vi "FTW-Example-ExpressionEvaluation.vi"() -> ()   [LabVIEW 2013]
uses:
  src/core/expression/FTW-Expr-BooleanExpressionResult.ctl
panel:
  out "All expectations satisfied?":bool=TRUE
  out "Tokenized Outputs":T2(array[cluster]) {"Compile Time" format="%.6fsec"; "Execute Time" format="%.6fsec"}
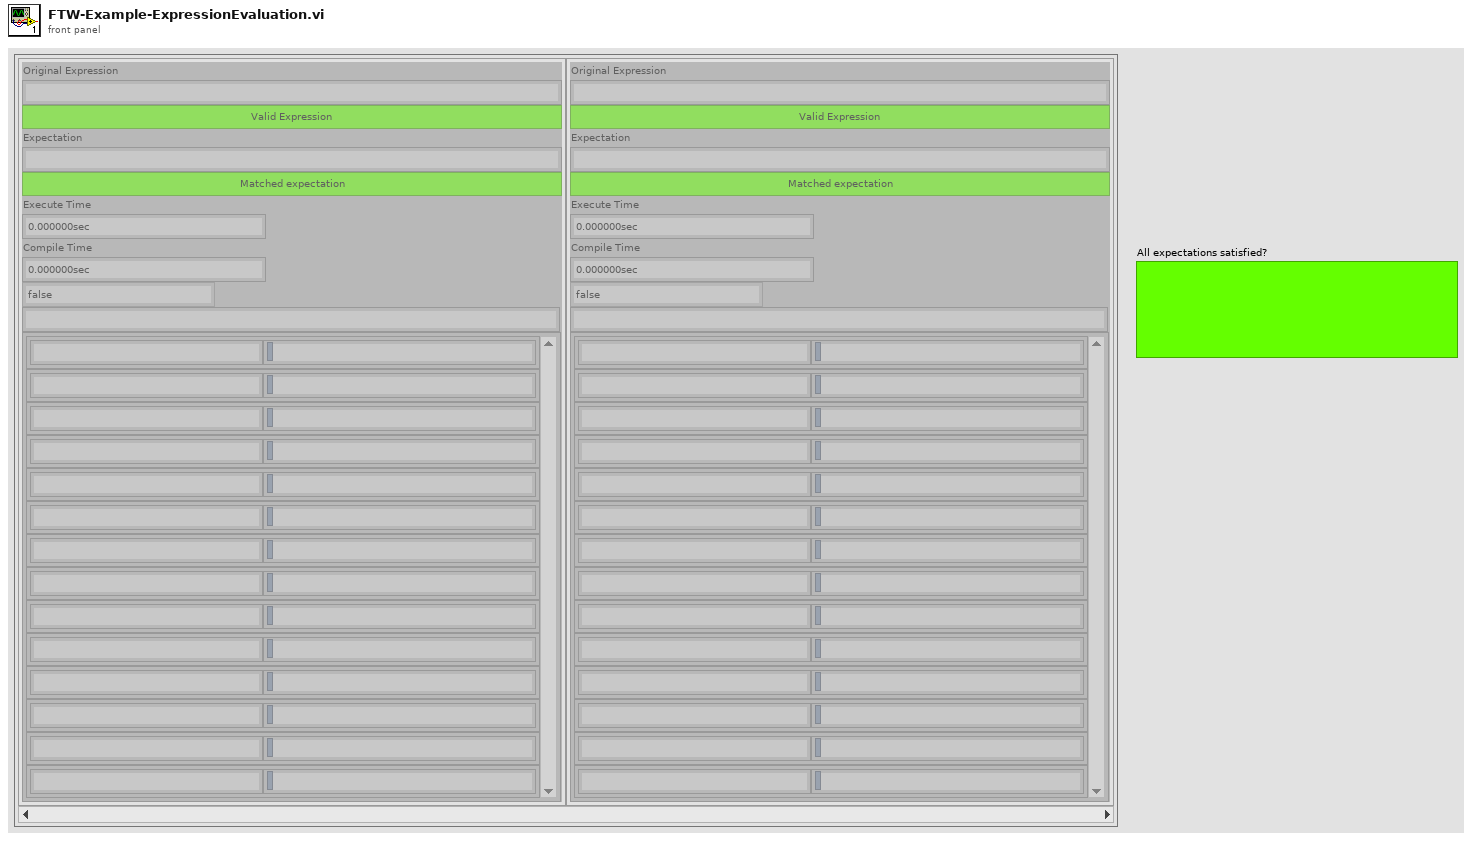
[diagram p1: front panel]
types:
  T1 = typedef "FTW-Expr-BooleanExpressionResult.ctl" = enum16{"false", "true", "inconclusive"}
  T2 = cluster{"Original Expression":string, "Valid?":bool, "Expectation":string, "Expectation satisfied?":bool, "Execute Time":dbl, "Compile Time":dbl, "Result":T1, "Error":string, "Tokens":cluster{string, string}[]}[]
  T3 = cluster{"Expression":string, "Expectation":string}[]
  T4 = cluster{"Expression":string, "Status OK?":bool, "Expectation":string, bool, "Total Time":dbl, "Compile Time":dbl, "Result":T1, "source":string, "Reverse Polish Notation Token Stack":cluster{string, string}[]}
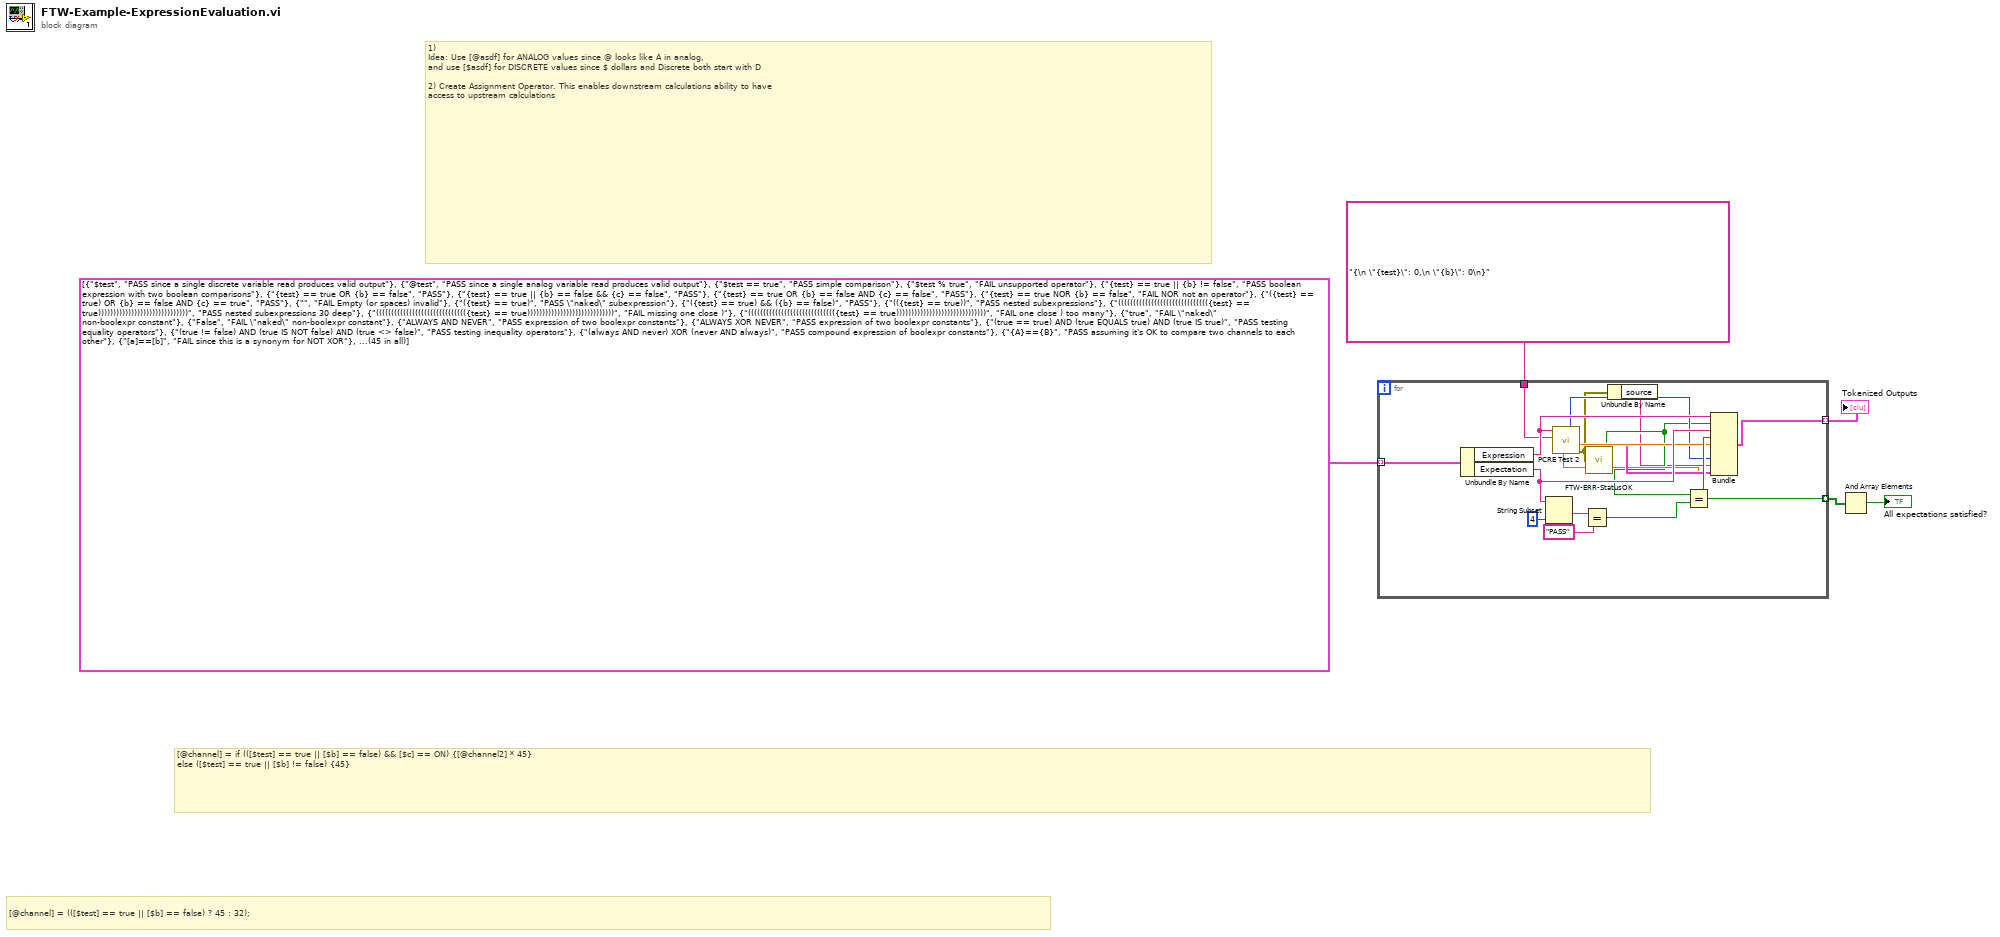
[diagram p0: block diagram]
diagram:
  # "[@channel] = (([$test] == true || [$b] == false) ? 45 : 32);"
  # "[@channel] = if (([$test] == true || [$b] == false) && [$c] == ON) {[@channel2] * 45}\nelse ([$test] == true || [$b] != false) {45}"
  # "1)\nIdea: Use [@asdf] for ANALOG values since @ looks like A in analog,\nand use [$asdf] for DISCRETE values since $ dollars and Discrete both start with D\n\n2) Create Assignment Operator. This enables downstream calculations ability to have\naccess to upstream calculations"
  n1 = for {
    tunnel: T3 [{"Expression"="$test", "Expectation"="PASS since a single discrete variable read produces valid output"}, {"Expression"="@test", "Expectation"="PASS since a single analog variable read produces valid output"}, {"Expression"="$test == true", "Expectation"="PASS simple comparison"}, {"Expression"="$test % true", "Expectation"="FAIL unsupported operator"}, {"Expression"="{test} == true || {b} != false", "Expectation"="PASS boolean expression with two boolean comparisons"}, {"Expression"="{test} == true OR {b} == false", "Expectation"="PASS"}, {"Expression"="{test} == true || {b} == false && {c} == false", "Expectation"="PASS"}, {"Expression"="{test} == true OR {b} == false AND {c} == false", "Expectation"="PASS"}, {"Expression"="{test} == true NOR {b} == false", "Expectation"="FAIL NOR not an operator"}, {"Expression"="({test} == true) OR {b} == false AND {c} == true", "Expectation"="PASS"}, {"Expression"="", "Expectation"="FAIL Empty (or spaces) invalid"}, {"Expression"="({test} == true)", "Expectation"="PASS \"naked\" subexpression"}, {"Expression"="({test} == true) && ({b} == false)", "Expectation"="PASS"}, {"Expression"="(({test} == true))", "Expectation"="PASS nested subexpressions"}, {"Expression"="(((((((((((((((((((((((((((((({test} == true))))))))))))))))))))))))))))))", "Expectation"="PASS nested subexpressions 30 deep"}, {"Expression"="(((((((((((((((((((((((((((((({test} == true)))))))))))))))))))))))))))))", "Expectation"="FAIL missing one close )"}, {"Expression"="((((((((((((((((((((((((((((({test} == true))))))))))))))))))))))))))))))", "Expectation"="FAIL one close ) too many"}, {"Expression"="true", "Expectation"="FAIL \"naked\" non-boolexpr constant"}, {"Expression"="False", "Expectation"="FAIL \"naked\" non-boolexpr constant"}, {"Expression"="ALWAYS AND NEVER", "Expectation"="PASS expression of two boolexpr constants"}, {"Expression"="ALWAYS XOR NEVER", "Expectation"="PASS expression of two boolexpr constants"}, {"Expression"="(true == true) AND (true EQUALS true) AND (true IS true)", "Expectation"="PASS testing equality operators"}, {"Expression"="(true != false) AND (true IS NOT false) AND (true <> false)", "Expectation"="PASS testing inequality operators"}, {"Expression"="(always AND never) XOR (never AND always)", "Expectation"="PASS compound expression of boolexpr constants"}, {"Expression"="{A}=={B}", "Expectation"="PASS assuming it's OK to compare two channels to each other"}, {"Expression"="[a]==[b]", "Expectation"="FAIL since this is a synonym for NOT XOR"}, {"Expression"="[a]!=[b]", "Expectation"="PASS since this is a synonym for XOR"}, {"Expression"="[A] AND [B]", "Expectation"="PASS assuming, variables are boolexpr states"}, {"Expression"="{a} IS true for 3 sec", "Expectation"="SKIP PASS simple timer test"}, {"Expression"="{a} IS true for 3min", "Expectation"="SKIP PASS no space between timer value and unit"}, {"Expression"="{a} IS true for 3", "Expectation"="SKIP FAIL no timer units"}, {"Expression"="{a} IS true   for minute", "Expectation"="SKIP FAIL no timer value"}, {"Expression"="{a} == true || [b] AND [c]", "Expectation"="PASS"}, {"Expression"="alwaysornever", "Expectation"="FAIL no word boundary on neither operator nor constants"}, {"Expression"="always||never", "Expectation"="PASS even though no spaces, the symbolic operator makes a word boundary"}, {"Expression"="(([a]&&[b]) OR ([c]&&[d])) AND (([e]&&[f]) OR ([g]&&[h]))", "Expectation"="PASS compound expression"}, {"Expression"="[a] (AND [b])", "Expectation"="FAIL improper placement of parentheses"}, {"Expression"="([a])([b])", "Expectation"="FAIL no operator between scopes"}, {"Expression"="([a])                   or                 ([b])", "Expectation"="PASS goofy amount of space"}, {"Expression"="NOT ALWAYS", "Expectation"="PASS the inversion of a boolexpr constant"}, {"Expression"="NOT [a] || [b]", "Expectation"="PASS even though it could use some parentheses for clarity, this is valid"}, {"Expression"="NOT ([a] || [b])", "Expectation"="PASS"}, {"Expression"="(NOT [a]) || [b]", "Expectation"="PASS"}, {"Expression"="[a] && ![b]", "Expectation"="PASS"}, {"Expression"="IMMEDIATELY", "Expectation"="PASS this is a synonym for ALWAYS"}] -> [w22] mode=indexing
    tunnel: [w16] -> w4 mode=indexing
    tunnel: [w14] -> w3 mode=indexing
    tunnel: "{\n \"{test}\": 0,\n \"{b}\": 0\n}" ("Values Table") -> [w10]
    n2 = Unbundle By Name(w22) -> ("Expression"=w17:string, "Expectation"=w15:string)
    n3 = String Subset(string=w15, length (rest)=4 ("length (rest)")) -> (substring=w20:string)  [unwired: 1 in]
    n4 = call "PCRE Test 2.vi"("Values Table"=w10, "Expression In"=w17) -> ("error out"=w7:errorcluster, "Reverse Polish Notation Token Stack"=w12:cluster{string, string}[], "Total Time"=w13:dbl, "Result"=w9:T1, "Compile Time"=w11:dbl)  [unwired: 5 in]
    n5 = Equal?(x=w20, y="PASS") -> (x = y?=w18:bool)
    n6 = call "FTW-ERR-StatusOK.vi"("error to check"=w7) -> ("Status OK?"=w8:bool)
    n7 = Unbundle By Name(w7) -> ("source"=w6:string)
    n8 = Equal?(x=w8, y=w18) -> (x = y?=w14:bool)
    n9 = Bundle("Expression"=w17, "Status OK?"=w8, "Expectation"=w15, w14, "Total Time"=w13, "Compile Time"=w11, "Result"=w9, "source"=w6, "Reverse Polish Notation Token Stack"=w12) -> (w16:T4)  [unwired: 1 in]
  }
  "Tokenized Outputs" <- w4
  n10 = And Array Elements(Boolean array=w3) -> (logical AND=→"All expectations satisfied?":bool)
